vi "young_serialcomm.vi"(7 "Reset Accum.":bool, 8 "Error In":errorcluster, 9 "Reset Code":string, 10 "Poll Code":string="MA!", 11 "Resource Name":refnum<visa-resource-name>) -> (0 "Error Out":errorcluster, 1 "Success":bool, 3 "Poll Response":string)   [LabVIEW 2018]
uses:
  <vilib>/Instr/_visa.llb/VISA Configure Serial Port (Instr).vi
panel:
  in  "byte count":u32
  out "Serial Settings:Number of Bytes at Serial Port":u32
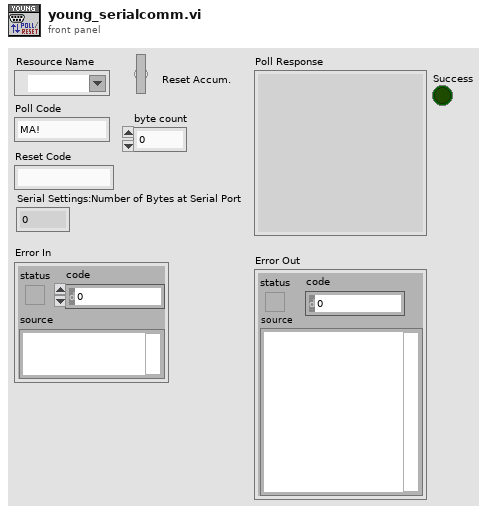
[diagram p1: front panel]
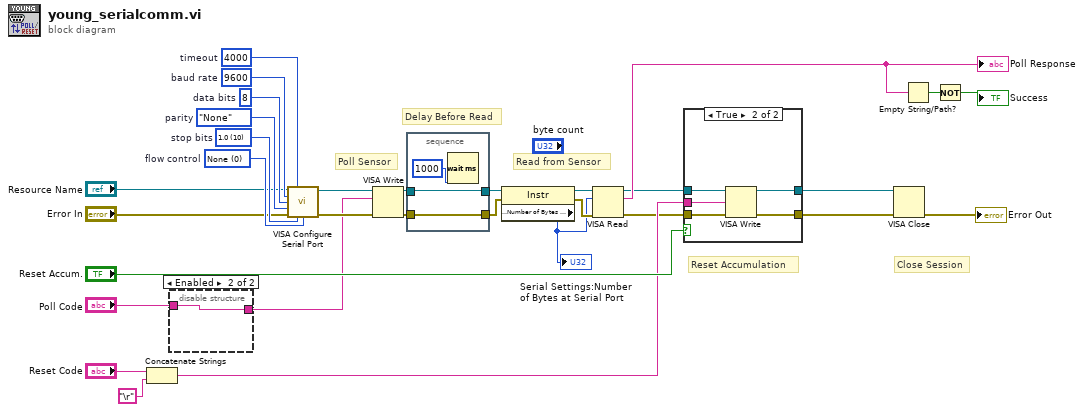
[diagram p0: block diagram]
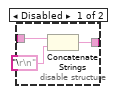
[diagram p2: hidden frame]
diagram:
  w21 = u16 0 items=["None", "XON/XOFF", "RTS/CTS", "XON/XOFF & RTS/CTS", "DTR/DSR", "XON/XOFF & DTR/DSR"]  # flow control
  w22 = u16 10 items=["1.0"=10, "1.5"=15, "2.0"=20]  # stop bits
  w26 = u32 4000  # timeout
  w23 = enum16{"None", "Odd", "Even", "Mark", "Space"}."None"  # parity
  w24 = u16 8  # data bits
  w25 = u32 9600  # baud rate
  # "Reset Accumulation"
  # "Delay Before Read"
  # "Read from Sensor"
  # "Poll Sensor"
  # "Close Session"
  n1 = Concatenate Strings("Reset Code", "\r") -> (w15:string)
  n2 = disable-structure shown="Enabled" {
    disable-tunnel: [w33 w35] -> w16
    disable-tunnel: "Poll Code" -> [w32 w35]
    frame Disabled {
      n3 = Concatenate Strings(w32, "\r\n") -> (w33:string)
    }
    frame Enabled {
    }
  }
  n4 = call-poly "VISA Configure Serial Port"("VISA resource name"="Resource Name", "timeout (10sec)"=w26, "baud rate (9600)"=w25, "data bits (8)"=w24, "parity (0:none)"=w23, "error in (no error)"="Error In", "stop bits (10: 1 bit)"=w22, "flow control (0:none)"=w21) -> ("VISA resource name out"=w29:refnum<visa-resource-name>, "error out"=w28:errorcluster)  [unwired: 1 in, 5 out]
  n5 = VISA Write(VISA resource name=w29, write buffer=w16, error in (no error)=w28) -> (VISA resource name out=w4:refnum<visa-resource-name>, error out=w2:errorcluster)  [unwired: 1 out]
  n6 = stacked-sequence {
    tunnel: w2 -> [w38]
    tunnel: [w38] -> w3
    tunnel: w4 -> [w37]
    tunnel: [w37] -> w5
    frame #0 {
      n7 = Wait (ms)(milliseconds to wait=u32 1000 ("delay before read (ms)")) -> ()  [unwired: 1 out]
    }
  }
  n8 = property class="Instr"(reference=w5, error in=w3) -> (reference out=w6:refnum<visa-resource-name>, error out=w7:errorcluster, "Serial Settings:Number of Bytes at Serial Port"=w1:u32)
  "Serial Settings:Number of Bytes at Serial Port" <- w1
  n9 = VISA Read(VISA resource name=w6, byte count=w1, error in (no error)=w7) -> (VISA resource name out=w8:refnum<visa-resource-name>, read buffer=w12:string, error out=w9:errorcluster)  [unwired: 1 out]
  "Poll Response" <- w12
  n10 = case shown="True" "Reset Accum." {
    tunnel: [w40 w43] -> w30
    tunnel: w8 -> [w40 w44]
    tunnel: [w39 w42] -> w31
    tunnel: w9 -> [w39 w45]
    tunnel: w15 -> [_ w41]
    frame False {
    }
    frame True {
      n11 = VISA Write(VISA resource name=w44, write buffer=w41, error in (no error)=w45) -> (VISA resource name out=w43:refnum<visa-resource-name>, error out=w42:errorcluster)  [unwired: 1 out]
    }
  }
  n12 = VISA Close(VISA resource name=w30, error in (no error)=w31) -> (error out=→"Error Out":errorcluster)
  n13 = Empty String/Path?(string/path=w12) -> (empty?=w11:bool)
  n14 = Not(x=w11) -> (.not. x?=→"Success":bool)
